vi "GetAllSerialComm.vi"(0 "VISA Address":string, 1 "reference":refnum<vi>) -> (2 "List":string[](array[string]), 3 "new?":bool, 4 "names":string[](array[string]))   [LabVIEW 2014]
panel:
  out "Array":string[](array[string])
  out "find list":string[](array[string])
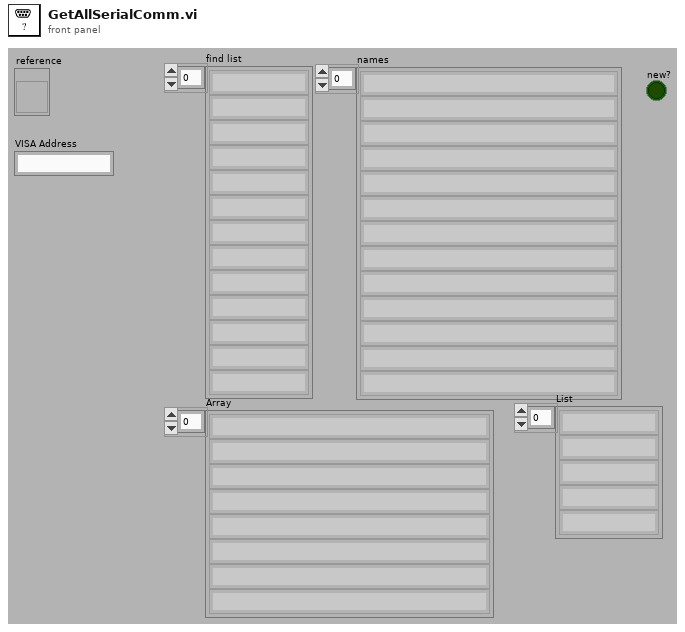
[diagram p1: front panel]
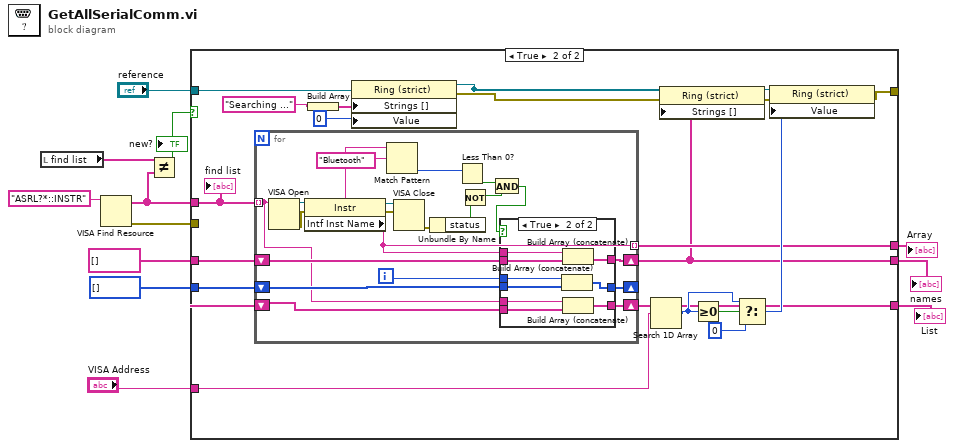
[diagram p0: block diagram]
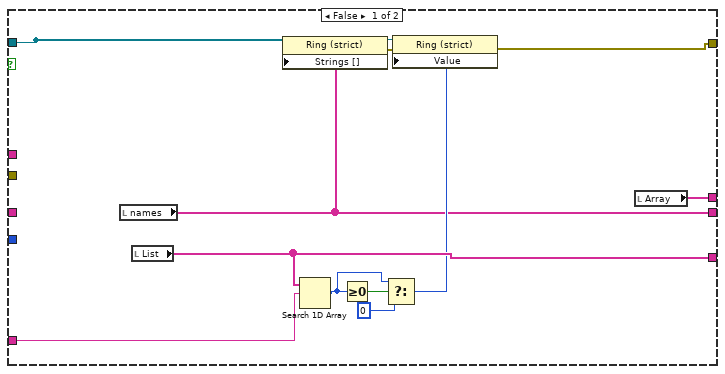
[diagram p2: hidden frame]
diagram:
  n1 = local read "find list"() -> (w6:string[])
  n2 = VISA Find Resource(11:"ASRL?*::INSTR" ("expression (\"?*\")")) -> (0:w2:errorcluster, 3:w7:string[])  [unwired: 2 in, 1 out]
  n3 = Not Equal?(x=w6, y=w7) -> (x != y?=w1:bool)
  "new?" <- w1
  n4 = case shown="True" w1 {
    tunnel: string[] [] -> [_ w38]
    tunnel: "VISA Address" -> [w15 w37]
    tunnel: i32[] [] -> [_ w36]
    tunnel: "reference" -> [w21 w26]
    tunnel: [w20 w34] -> _
    tunnel: w7 -> [_ w33]
    tunnel: [w23 w32] -> w5
    tunnel: [w13 w31] -> w4
    tunnel: [w16 w30] -> w3
    tunnel: w2 -> [_ _]
    frame False {
      n5 = local read "names"() -> (w13:string[])
      n6 = local read "List"() -> (w16:string[])
      n7 = property on="Property Node" class="Ring (strict)"(reference=w21, "Strings []"=w13) -> (error out=w22:errorcluster)  [unwired: 1 in, 1 out]
      n8 = Search 1D Array(1D array=w16, element=w15) -> (index of element=w18:i32)  [unwired: 1 in]
      n9 = Greater Or Equal To 0?(x=w18) -> (x >= 0?=w17:bool)
      n10 = Select(t=w18, s=w17, f=0) -> (s? t:f=w14:i32)
      n11 = property class="Ring (strict)"(reference=w21, error in=w22, "Value"=w14) -> (error out=w20:errorcluster)  [unwired: 1 out]
      n12 = local read "Array"() -> (w23:string[])
    }
    frame True {
      n13 = for {
        tunnel: w33 -> [w52] mode=indexing
        shift-right: [w58] -> w31
        shift-left: w38 -> [w57]
        shift-right: [w55] -> _
        shift-left: w36 -> [w54]
        tunnel: [w50] -> w32 mode=indexing
        shift-right: [w53] -> w30
        shift-left: w38 -> [w51]
        i -> [w56]
        n14 = VISA Open(VISA resource name=w52) -> (VISA resource name=w62:refnum<visa-resource-name>, error out=w60:errorcluster)  [unwired: 4 in]
        n15 = property class="Instr"(reference=w62, error in=w60) -> (reference out=w61:refnum<visa-resource-name>, error out=w59:errorcluster, "Intf Inst Name"=w50:string)
        n16 = Match Pattern(string=w50, regular expression="Bluetooth" ("task")) -> (offset past match=w48:i32)  [unwired: 1 in, 3 out]
        n17 = VISA Close(VISA resource name=w61, error in (no error)=w59) -> (error out=w46:errorcluster)
        n18 = Unbundle By Name(w46) -> ("status"=w45:bool)
        n19 = Less Than 0?(x=w48) -> (x < 0?=w47:bool)
        n20 = Not(x=w45) -> (.not. x?=w44:bool)
        n21 = And(x=w47, y=w44) -> (x .and. y?=w43:bool)
        n22 = case shown="True" w43 {
          tunnel: w50 -> [_ w67]
          tunnel: [w65 w74] -> w58
          tunnel: w57 -> [w65 w73]
          tunnel: w56 -> [_ w66]
          tunnel: [w64 w71] -> w55
          tunnel: w54 -> [w64 w72]
          tunnel: [w63 w70] -> w53
          tunnel: w52 -> [_ w69]
          tunnel: w51 -> [w63 w68]
          frame False {
          }
          frame True {
            n23 = Build Array (concatenate)(w66, w72) -> (w71:i32[])
            n24 = Build Array (concatenate)(w67, w73) -> (w74:string[])
            n25 = Build Array (concatenate)(w69, w68) -> (w70:string[])
          }
        }
      }
      n26 = Build Array("Searching ..." ("task")) -> (w28:string[])
      n27 = property on="Property Node" class="Ring (strict)"(reference=w26, "Strings []"=w28, "Value"=0) -> (reference out=w25:refnum<vi>, error out=w24:errorcluster)  [unwired: 1 in]
      n28 = Search 1D Array(1D array=w30, element=w37) -> (index of element=w40:i32)  [unwired: 1 in]
      n29 = property on="Property Node" class="Ring (strict)"(reference=w25, error in=w24, "Strings []"=w31) -> (error out=w35:errorcluster)  [unwired: 1 out]
      n30 = Greater Or Equal To 0?(x=w40) -> (x >= 0?=w39:bool)
      n31 = Select(t=w40, s=w39, f=0) -> (s? t:f=w42:i32)
      n32 = property class="Ring (strict)"(reference=w25, error in=w35, "Value"=w42) -> (error out=w34:errorcluster)  [unwired: 1 out]
      "find list" <- w33
    }
  }
  "Array" <- w5
  "names" <- w4
  "List" <- w3
